vi "Build_Auth_URL.vi"(8 "error in (no error)":errorcluster, 10 "Application":T1, 11 "OAuth in":refnum<class "OAuth.lvclass">) -> (0 "error out":errorcluster, 3 "OAuth out":refnum<class "OAuth.lvclass">)   [LabVIEW 2016, in "OAuth.lvclass"]
uses:
  OAuth.lvclass
  scope_needed.ctl
  OAuth.lvclass/OAuth.ctl
  <vilib>/addons/_JKI.lib/REST Client/classes/REST Client/REST Client.lvclass
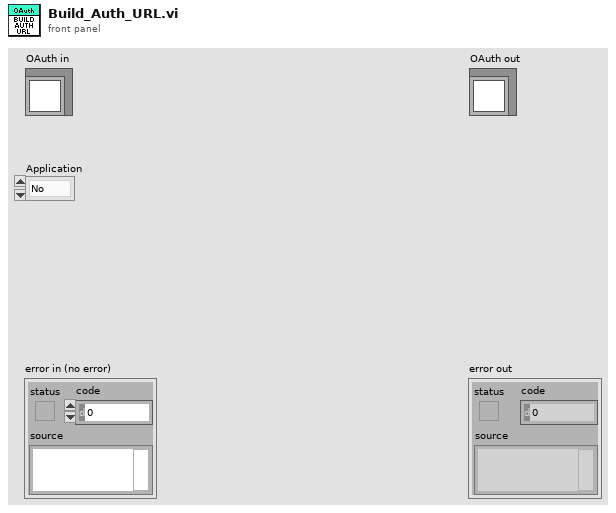
[diagram p1: front panel]
types:
  T1 = typedef "scope_needed.ctl" = enum16{"No", "Yes"}
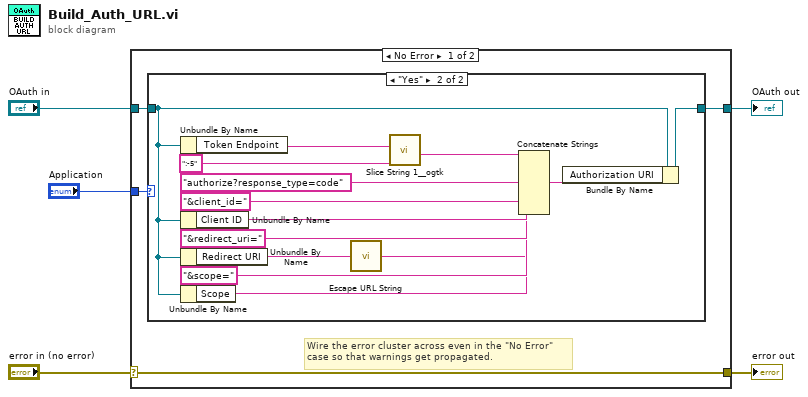
[diagram p0: block diagram]
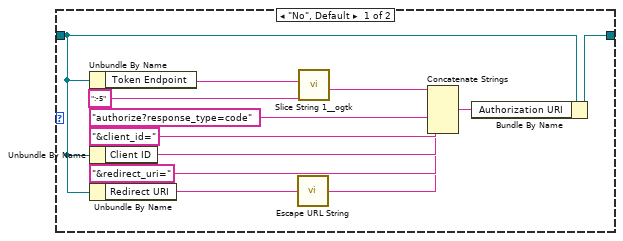
[diagram p2: hidden frame]
diagram:
  n1 = case shown="No Error" "error in (no error)" {
    selector: "error in (no error)" -> [w9 w37]
    tunnel: [w9 w37] -> w4
    tunnel: [w8 w36] -> w2
    tunnel: "OAuth in" -> [w7 w36]
    tunnel: "Application" -> [w6 _]
    frame No Error {
      # "Wire the error cluster across even in the \"No Error\"\ncase so that warnings get propagated."
      n2 = case shown="\"Yes\"" w6 {
        tunnel: [w18 w32] -> w8
        tunnel: w7 -> [w16 w26]
        frame "No", Default {
          n3 = Unbundle By Name(w16) -> ("Token Endpoint"=w15:string)
          n4 = Unbundle By Name(w16) -> ("Client ID"=w12:string)
          n5 = Unbundle By Name(w16) -> ("Redirect URI"=w14:string)
          n6 = call <vilib>:"Escape URL String.vi"("Unescaped URL string in"=w14) -> ("Escaped URL string out"=w10:string)
          n7 = call <userlib>:"Slice String 1__ogtk.vi"("Subset (i:j)"=":-5", "String"=w15) -> ("Substring (String[i:j])"=w21:string)  [unwired: 7 in]
          n8 = Concatenate Strings(w21, "authorize?response_type=code", "&client_id=", w12, "&redirect_uri=", w10) -> (w17:string)
          n9 = Bundle By Name(cluster=w16, "Authorization URI"=w17) -> (w18:refnum<class "OAuth.lvclass">)
        }
        frame "Yes" {
          n10 = Unbundle By Name(w26) -> ("Token Endpoint"=w30:string)
          n11 = Unbundle By Name(w26) -> ("Client ID"=w28:string)
          n12 = Unbundle By Name(w26) -> ("Redirect URI"=w23:string)
          n13 = Unbundle By Name(w26) -> ("Scope"=w24:string)
          n14 = call <vilib>:"Escape URL String.vi"("Unescaped URL string in"=w23) -> ("Escaped URL string out"=w22:string)
          n15 = call <userlib>:"Slice String 1__ogtk.vi"("Subset (i:j)"=":-5", "String"=w30) -> ("Substring (String[i:j])"=w35:string)  [unwired: 7 in]
          n16 = Concatenate Strings(w35, "authorize?response_type=code", "&client_id=", w28, "&redirect_uri=", w22, "&scope=", w24) -> (w31:string)
          n17 = Bundle By Name(cluster=w26, "Authorization URI"=w31) -> (w32:refnum<class "OAuth.lvclass">)
        }
      }
    }
    frame Error {
    }
  }
  "error out" <- w4
  "OAuth out" <- w2
